vi "CTR Start.vi"(8 "error in (no error)":errorcluster, 11 "NI Multifunction IO in":refnum<class "NI Multifunction IO.lvclass">) -> (0 "error out":errorcluster, 3 "NI Multifunction IO out":refnum<class "NI Multifunction IO.lvclass">)   [LabVIEW 2020, in "NI Multifunction IO.lvlib" / "NI Multifunction IO.lvclass"]
uses:
  NI Multifunction IO.lvclass
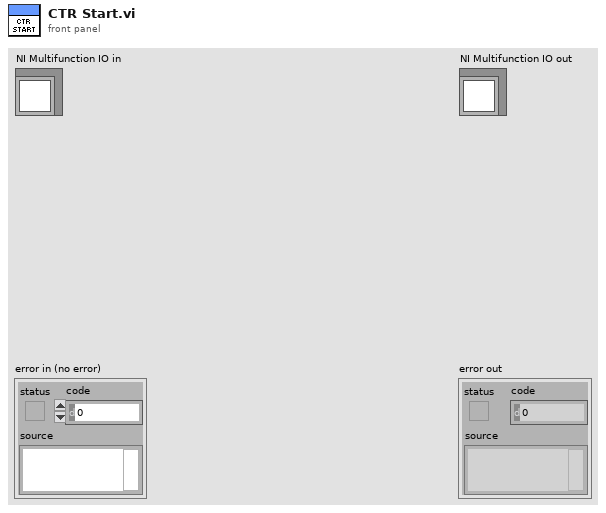
[diagram p1: front panel]
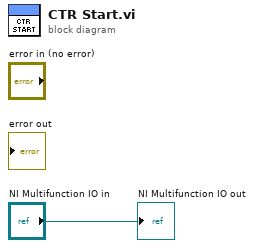
[diagram p0: block diagram]
diagram:
  "NI Multifunction IO out" <- "NI Multifunction IO in"
